vi "focusKnobMove.vi"(1 "position (10^-4 m)":i32) -> ()   [LabVIEW 2017]
uses:
  globalDevices.vi
panel:
  out "read buffer":string
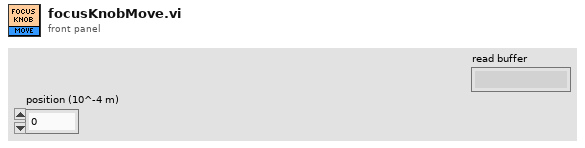
[diagram p1: front panel]
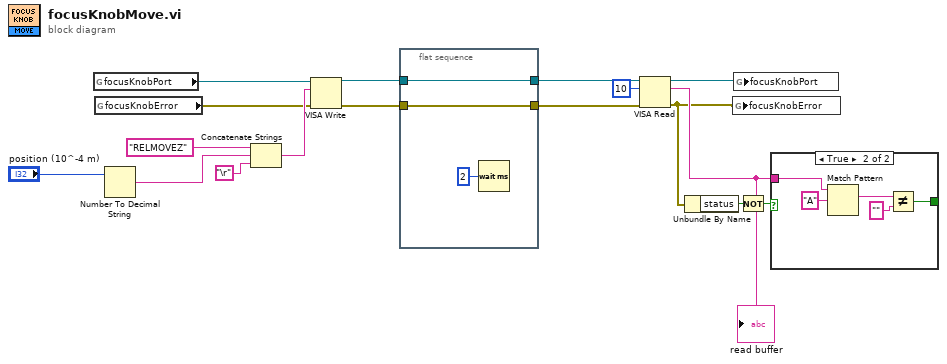
[diagram p0: block diagram]
diagram:
  n1 = global read "globalDevices.vi" "focusKnobPort"() -> (w17:refnum<visa-resource-name>)
  n2 = global read "globalDevices.vi" "focusKnobError"() -> (w1:errorcluster)
  n3 = Number To Decimal String(number="position (10^-4 m)") -> (decimal integer string=w14:string)  [unwired: 1 in]
  n4 = Concatenate Strings("RELMOVEZ" ("string"), w14, "\r") -> (w12:string)
  n5 = VISA Write(VISA resource name=w17, write buffer=w12, error in (no error)=w1) -> (VISA resource name out=w5:refnum<visa-resource-name>, error out=w3:errorcluster)  [unwired: 1 out]
  n6 = flat-sequence {
    tunnel: w5 -> [w20]
    tunnel: [w20] -> w4
    tunnel: [w19] -> w2
    tunnel: w3 -> [w19]
    frame #0 {
      n7 = Wait (ms)(milliseconds to wait=u32 2) -> ()  [unwired: 1 out]
    }
  }
  n8 = VISA Read(VISA resource name=w4, byte count=u32 10, error in (no error)=w2) -> (VISA resource name out=w7:refnum<visa-resource-name>, read buffer=w8:string, error out=w6:errorcluster)  [unwired: 1 out]
  "read buffer" <- w8
  n9 = Unbundle By Name(w6) -> ("status"=w10:bool)
  n10 = global write "globalDevices.vi" "focusKnobError"(w6) -> ()
  n11 = global write "globalDevices.vi" "focusKnobPort"(w7) -> ()
  n12 = Not(x=w10) -> (.not. x?=w9:bool)
  n13 = case shown="True" w9 {
    selector: w9 -> [w21 _]
    tunnel: w8 -> [_ w26]
    tunnel: [w21 w22] -> _
    frame False {
    }
    frame True {
      n14 = Match Pattern(string=w26, regular expression="A") -> (match substring=w24:string)  [unwired: 1 in, 3 out]
      n15 = Not Equal?(x=w24, y="") -> (x != y?=w22:bool)
    }
  }
